vi "I32toString_FixLength.vi"(1 "I32":i32, 6 "Length (Nb Char)":u8) -> (15 "String OUT":string)   [LabVIEW 2022 SP3, in "stillnessHelper.lvclass"]
uses:
  stillnessHelper.lvclass
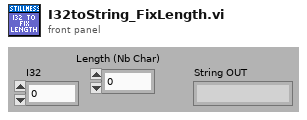
[diagram p1: front panel]
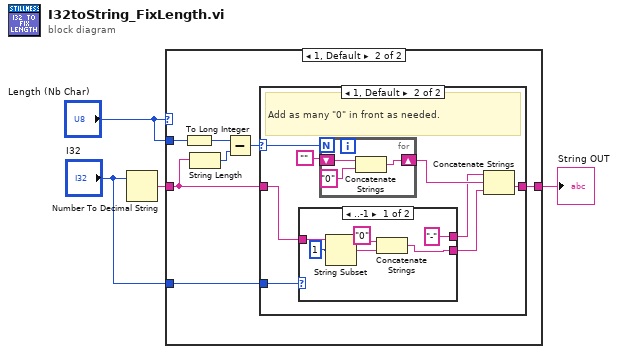
[diagram p0: block diagram]
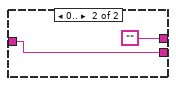
[diagram p4: hidden frame]
diagram:
  n1 = Number To Decimal String(number="I32") -> (decimal integer string=w3:string)  [unwired: 1 in]
  n2 = case shown="1, Default" "Length (Nb Char)" {
    tunnel: [w5 w8] -> w4
    tunnel: w3 -> [w5 w7]
    tunnel: "Length (Nb Char)" -> [_ w12]
    tunnel: "I32" -> [_ w6]
    frame 0 {
      # "Do Nothing"
    }
    frame 1, Default {
      n3 = To Long Integer(number=w12) -> (32bit integer=w10:i32)
      n4 = String Length(string=w7) -> (length=w11:i32)
      n5 = Subtract(x=w10, y=w11) -> (x-y=w9:i32)
      n6 = case shown="1, Default" w9 {
        selector: w9 -> [_ w21]
        tunnel: [w13 w19] -> w8
        tunnel: w7 -> [w13 w16]
        tunnel: w6 -> [_ w17]
        frame ..0 {
          # "The string lenght is equal or greater, so do nothing"
        }
        frame 1, Default {
          # "Add as many \"0\" in front as needed."
          n7 = case shown="..-1" w17 {
            tunnel: w16 -> [w27 w29]
            tunnel: [w22 w29] -> w15
            tunnel: ["-" ""] -> w14
            frame ..-1 {
              n8 = String Subset(string=w27, offset (0)=1) -> (substring=w24:string)  [unwired: 1 in]
              n9 = Concatenate Strings("0", w24) -> (w22:string)
            }
            frame 0.. {
            }
          }
          n10 = for {
            N: w21 -> [_]
            shift-right: [w31] -> w18
            shift-left: "" -> [w32]
            n11 = Concatenate Strings(w32, "0") -> (w31:string)
          }
          n12 = Concatenate Strings(w14, w18, w15) -> (w19:string)
        }
      }
    }
  }
  "String OUT" <- w4
